vi "Write Return DeviceID Array Msg.vi"(10 "Return DeviceID Array Msg":refnum<class "Return DeviceID Array Msg.lvclass">, 11 "SCADA in":refnum<class "EMS.lvclass">) -> (3 "SCADA out":refnum<class "EMS.lvclass">)   [LabVIEW 2018, in "EMS Core.lvlib" / "EMS.lvclass"]
uses:
  EMS.lvclass
  EMS Messages/Return DeviceID Array Msg/Return DeviceID Array Msg.lvclass
  EMS.lvclass/EMS.ctl
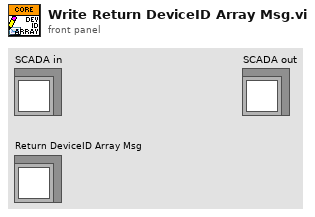
[diagram p1: front panel]
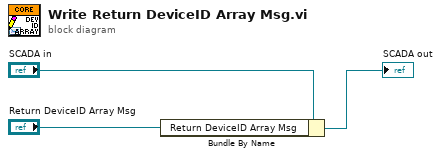
[diagram p0: block diagram]
diagram:
  n1 = Bundle By Name(cluster="SCADA in", "Return DeviceID Array Msg"="Return DeviceID Array Msg") -> (→"SCADA out":refnum<class "EMS.lvclass">)
